vi "Get_object_size_from_b.box.vi"(2 "Error In":errorcluster, 3 "Bounding rectangle for cage outline, pix":T1) -> (0 "Error Out":errorcluster, 1 "Object Size, pix":cluster{"W":dbl, "H":dbl})   [LabVIEW 2018, in "Cage Diagram.lvlib"]
uses:
  Cage Diagram.lvlib
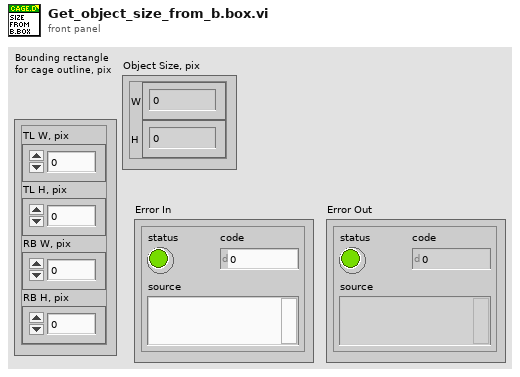
[diagram p1: front panel]
types:
  T1 = cluster{"TL W, pix":dbl, "TL H, pix":dbl, "RB W, pix":dbl, "RB H, pix":dbl}
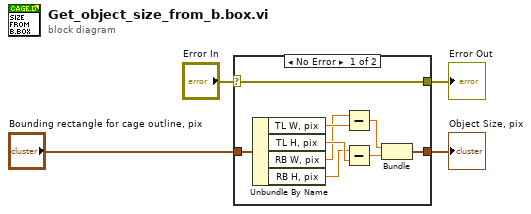
[diagram p0: block diagram]
diagram:
  n1 = case shown="No Error" "Error In" {
    selector: "Error In" -> [w5 w14]
    tunnel: "Bounding rectangle for cage outline, pix" -> [w9 _]
    tunnel: [w6 _] -> w3
    tunnel: [w5 w14] -> w1
    frame No Error {
      n2 = Unbundle By Name(w9) -> ("TL W, pix"=w11:dbl, "TL H, pix"=w13:dbl, "RB W, pix"=w10:dbl, "RB H, pix"=w12:dbl)
      n3 = Subtract(x=w10, y=w11) -> (x-y=w8:dbl)
      n4 = Subtract(x=w12, y=w13) -> (x-y=w7:dbl)
      n5 = Bundle(w8, w7) -> (w6:cluster{dbl, dbl})  [unwired: 1 in]
    }
    frame Error {
    }
  }
  "Object Size, pix" <- w3
  "Error Out" <- w1
